vi "lsl get session id.vi"(8 "error in (no error)":errorcluster, 11 "streaminfo":T1) -> (0 "error out":errorcluster, 3 "session ID":string)   [LabVIEW 2018, in "liblsl-LabVIEW.lvlib"]
doc: "extern LIBLSL_C_API const char *lsl_get_session_id(lsl_streaminfo info);"
uses:
  <userlib>/liblsl-LabVIEW/liblsl-LabVIEW.lvlib
  <userlib>/liblsl-LabVIEW/Custom Controls/lsl_streaminfo.ctl
  <userlib>/liblsl-LabVIEW/liblsl64.dll
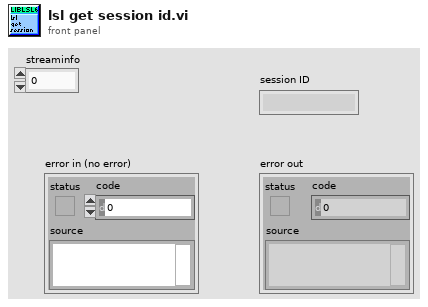
[diagram p1: front panel]
types:
  T1 = typedef "liblsl-LabVIEW.lvlib/lsl_streaminfo.ctl" = u64
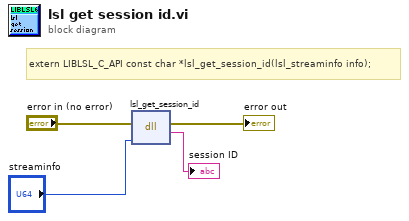
[diagram p0: block diagram]
diagram:
  # "extern LIBLSL_C_API const char *lsl_get_session_id(lsl_streaminfo info);"
  n1 = dll-call lib="C:/Program Files/National Instruments/LabVIEW 2018/user.lib/liblsl-LabVIEW/liblsl64.*" fn="lsl_get_session_id"(error in="error in (no error)", "info"="streaminfo") -> (error out=→"error out":errorcluster, "return type"=→"session ID":string)  [unwired: 3 in, 1 out]
